vi "Search Text File.vi"(10 "Subject Number":string, 11 "Spreadsheet String":string) -> (0 "SPARC Data":dbl[](array[numeric]), 1 "NMD Data":dbl[](array[numeric]), 2 "SPARC Data Text":string[](array[string]), 3 "NMD Data Text":string[](array[string]))   [LabVIEW 2021]
uses:
  <vilib>/Analysis/baseanly.llb/Mean (DBL).vi
  <vilib>/Analysis/NI_AALBase.lvlib
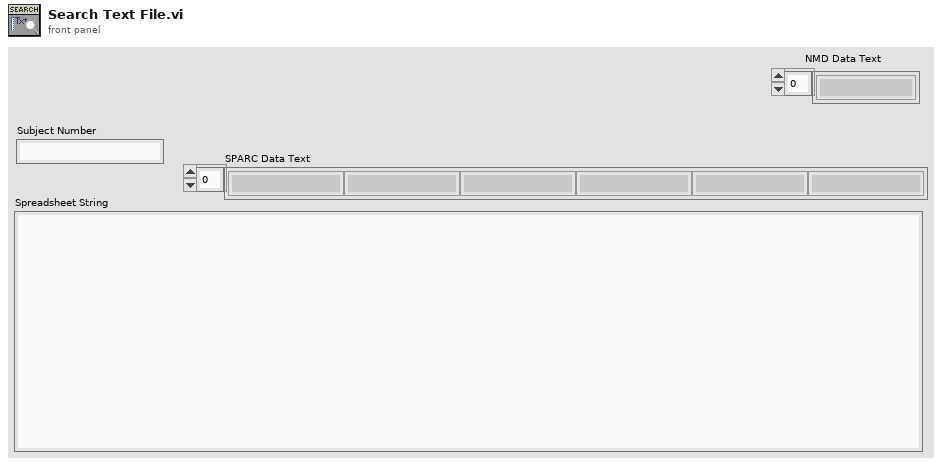
[diagram p1: front panel]
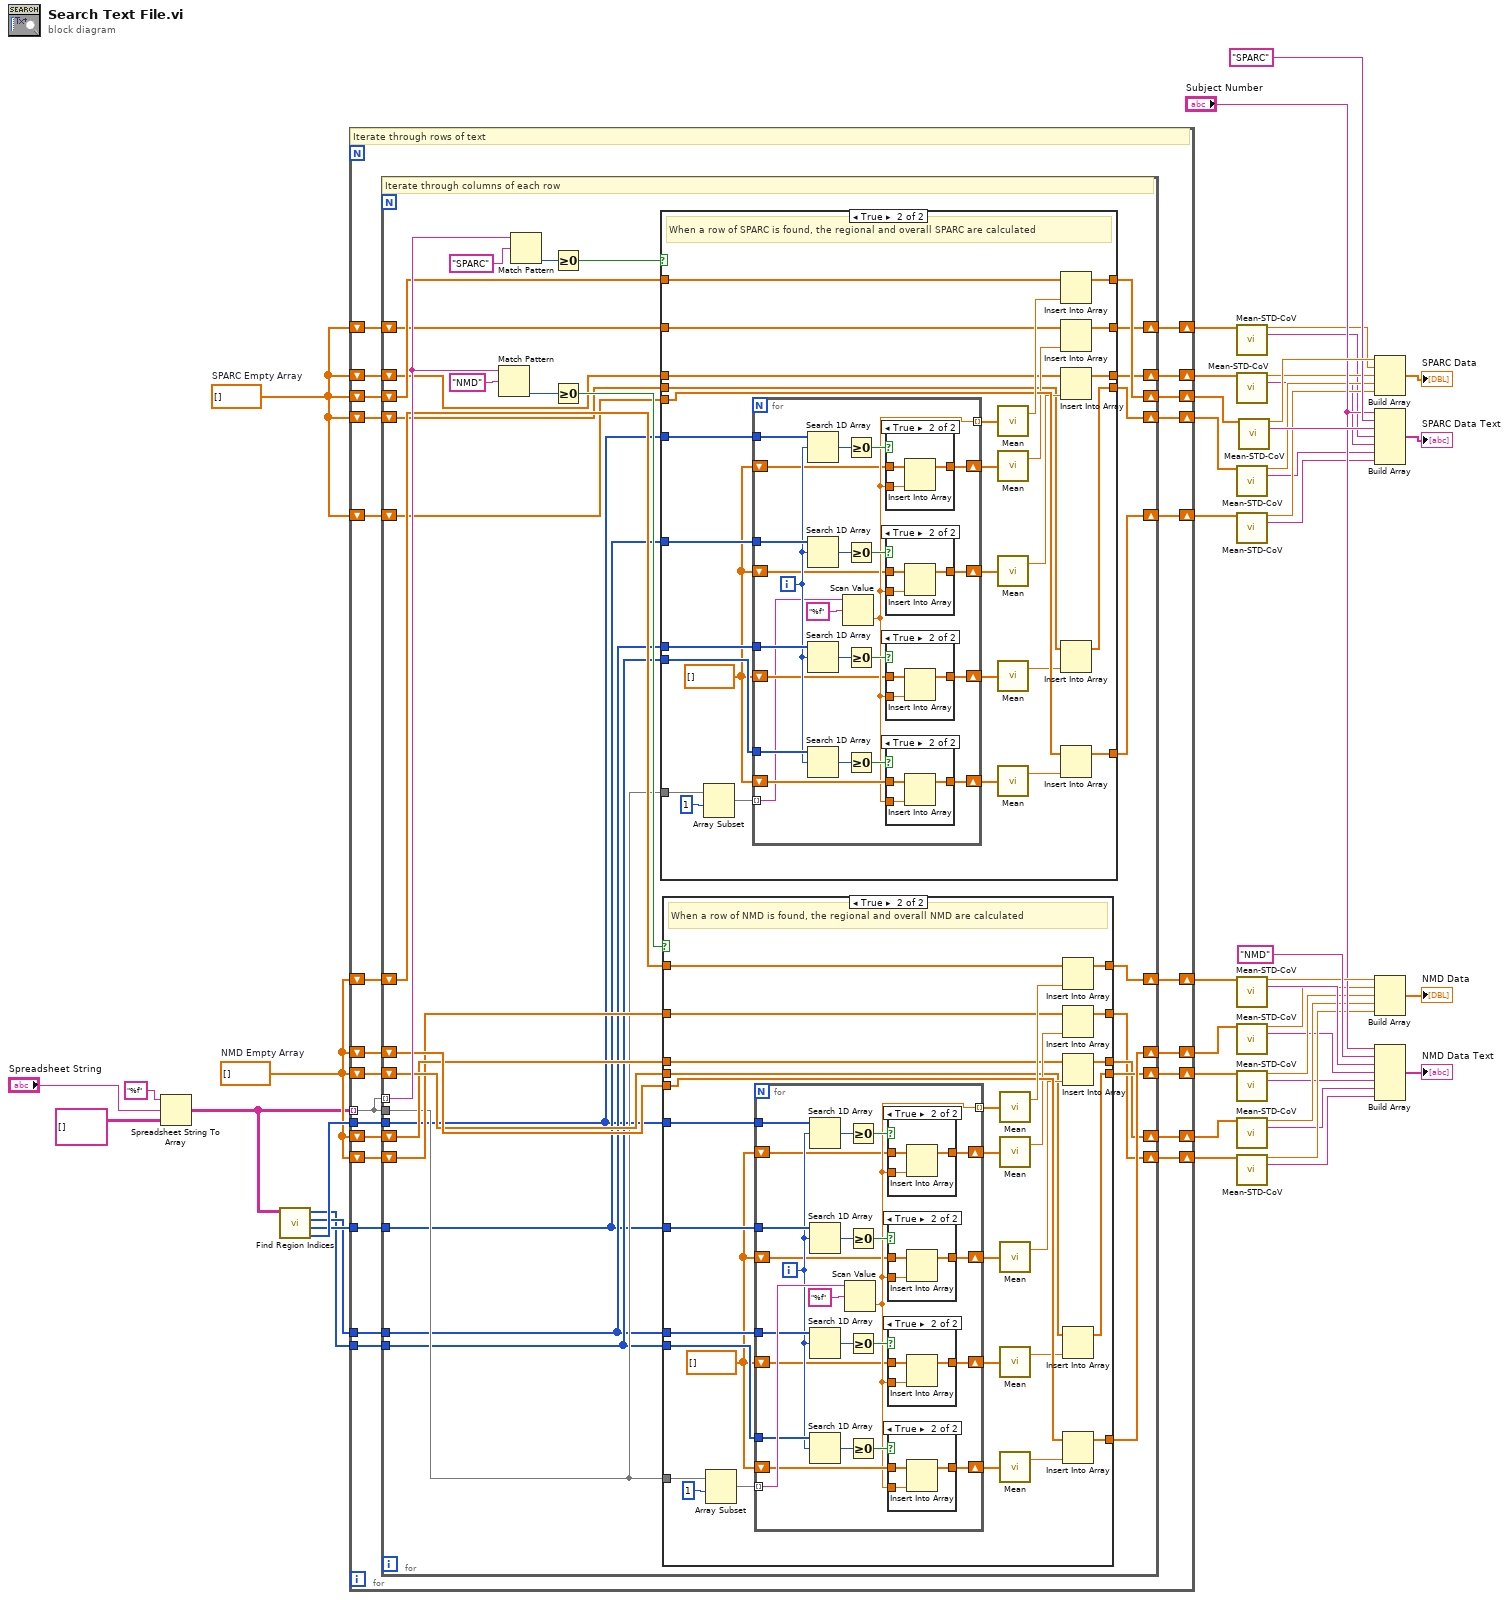
[diagram p0: block diagram]
diagram:
  w38 = dbl[] []  # SPARC Empty Array
  w39 = dbl[] []  # NMD Empty Array
  n1 = Spreadsheet String To Array(format string="%f", spreadsheet string="Spreadsheet String", array type (2D Dbl)=string[][] []) -> (array=w1:string[][])  [unwired: 1 in]
  n2 = call "Find Region Indices.vi"("Spreadsheet Array"=w1) -> ("UES Index"=w43:i32[], "Hypo Index"=w42:i32[], "Tongue Index"=w41:i32[], "Velo Index"=w40:i32[])  [unwired: 7 in]
  n3 = for {
    shift-right: [w71] -> w44
    shift-left: w39 -> [w72]
    shift-right: [w69] -> w31
    shift-left: w38 -> [w70]
    shift-right: [w67] -> w35
    shift-left: w39 -> [w68]
    tunnel: w43 -> [w66]
    tunnel: w42 -> [w65]
    tunnel: w41 -> [w64]
    tunnel: w40 -> [w63]
    tunnel: w1 -> [w62] mode=indexing
    shift-right: [w58] -> w34
    shift-left: w39 -> [w61]
    shift-right: [w57] -> w33
    shift-left: w39 -> [w60]
    shift-right: [w56] -> w32
    shift-left: w39 -> [w59]
    shift-right: [w48] -> w30
    shift-left: w38 -> [w52]
    shift-right: [w49] -> w29
    shift-left: w38 -> [w53]
    shift-right: [w50] -> w28
    shift-left: w38 -> [w54]
    shift-right: [w51] -> w27
    shift-left: w38 -> [w55]
    # "Iterate through rows of text"
    n4 = for {
      tunnel: w62 -> [w100] mode=indexing
      shift-right: [w98] -> w71
      shift-left: w72 -> [w99]
      shift-right: [w82] -> w69
      shift-left: w70 -> [w83]
      shift-right: [w95] -> w67
      shift-left: w68 -> [w96]
      tunnel: w66 -> [w84]
      tunnel: w65 -> [w85]
      tunnel: w64 -> [w86]
      tunnel: w63 -> [w87]
      tunnel: w62 -> [w88]
      shift-right: [w91] -> w58
      shift-left: w61 -> [w94]
      shift-right: [w90] -> w57
      shift-left: w60 -> [w93]
      shift-right: [w89] -> w56
      shift-left: w59 -> [w92]
      shift-right: [w74] -> w48
      shift-left: w52 -> [w78]
      shift-right: [w75] -> w49
      shift-left: w53 -> [w79]
      shift-right: [w76] -> w50
      shift-left: w54 -> [w80]
      shift-right: [w77] -> w51
      shift-left: w55 -> [w81]
      # "Iterate through columns of each row"
      n5 = Match Pattern(string=w100, regular expression="NMD" ("element")) -> (offset past match=w104:i32)  [unwired: 1 in, 3 out]
      n6 = Match Pattern(string=w100, regular expression="SPARC" ("element")) -> (offset past match=w103:i32)  [unwired: 1 in, 3 out]
      n7 = Greater Or Equal To 0?(x=w103) -> (x >= 0?=w73:bool)
      n8 = Greater Or Equal To 0?(x=w104) -> (x >= 0?=w97:bool)
      n9 = case shown="True" w73 {
        tunnel: w83 -> [w109 w135]
        tunnel: [w109 w133] -> w82
        tunnel: w88 -> [_ w132]
        tunnel: w87 -> [_ w131]
        tunnel: w86 -> [_ w128]
        tunnel: w85 -> [_ w129]
        tunnel: w84 -> [_ w130]
        tunnel: w81 -> [w108 w126]
        tunnel: [w108 w125] -> w77
        tunnel: w80 -> [w107 w116]
        tunnel: w79 -> [w106 w115]
        tunnel: w78 -> [w105 w114]
        tunnel: [w107 w113] -> w76
        tunnel: [w106 w112] -> w75
        tunnel: [w105 w111] -> w74
        frame False {
        }
        frame True {
          w123 = dbl[] []
          # "When a row of SPARC is found, the regional and overall SPARC are calculated"
          n10 = Array Subset(array=w132, index=1) -> (w110:string[])  [unwired: 1 in]
          n11 = for {
            tunnel: w110 -> [w138] mode=indexing
            tunnel: [w145] -> w136 mode=indexing
            tunnel: w131 -> [w160]
            tunnel: w130 -> [w159]
            tunnel: w129 -> [w158]
            tunnel: w128 -> [w157]
            shift-right: [w149] -> w127
            shift-left: w123 -> [w150]
            shift-right: [w141] -> w117
            shift-left: w123 -> [w142]
            shift-right: [w140] -> w119
            shift-left: w123 -> [w143]
            shift-right: [w139] -> w121
            shift-left: w123 -> [w144]
            i -> [w152]
            n12 = Search 1D Array(1D array=w159, element=w152) -> (index of element=w154:i32)  [unwired: 1 in]
            n13 = Search 1D Array(1D array=w158, element=w152) -> (index of element=w155:i32)  [unwired: 1 in]
            n14 = Search 1D Array(1D array=w157, element=w152) -> (index of element=w153:i32)  [unwired: 1 in]
            n15 = Search 1D Array(1D array=w160, element=w152) -> (index of element=w156:i32)  [unwired: 1 in]
            n16 = Scan Value(string=w138, format string="%f") -> (value=w145:dbl)  [unwired: 1 in, 1 out]
            n17 = Greater Or Equal To 0?(x=w154) -> (x >= 0?=w146:bool)
            n18 = Greater Or Equal To 0?(x=w155) -> (x >= 0?=w147:bool)
            n19 = Greater Or Equal To 0?(x=w153) -> (x >= 0?=w148:bool)
            n20 = Greater Or Equal To 0?(x=w156) -> (x >= 0?=w151:bool)
            n21 = case shown="True" w146 {
              tunnel: w142 -> [w162 w165]
              tunnel: w145 -> [_ w164]
              tunnel: [w162 w163] -> w141
              frame False {
              }
              frame True {
                n22 = Insert Into Array(array=w165, new element=w164) -> (w163:dbl[])  [unwired: 1 in]
              }
            }
            n23 = case shown="True" w147 {
              tunnel: w143 -> [w166 w169]
              tunnel: w145 -> [_ w168]
              tunnel: [w166 w167] -> w140
              frame False {
              }
              frame True {
                n24 = Insert Into Array(array=w169, new element=w168) -> (w167:dbl[])  [unwired: 1 in]
              }
            }
            n25 = case shown="True" w148 {
              tunnel: w144 -> [w170 w173]
              tunnel: w145 -> [_ w172]
              tunnel: [w170 w171] -> w139
              frame False {
              }
              frame True {
                n26 = Insert Into Array(array=w173, new element=w172) -> (w171:dbl[])  [unwired: 1 in]
              }
            }
            n27 = case shown="True" w151 {
              tunnel: w150 -> [w174 w177]
              tunnel: w145 -> [_ w176]
              tunnel: [w174 w175] -> w149
              frame False {
              }
              frame True {
                n28 = Insert Into Array(array=w177, new element=w176) -> (w175:dbl[])  [unwired: 1 in]
              }
            }
          }
          n29 = call-poly <vilib>:"Mean.vi"("X"=w136) -> ("mean"=w134:dbl)  [unwired: 1 out]
          n30 = call-poly <vilib>:"Mean.vi"("X"=w117) -> ("mean"=w118:dbl)  [unwired: 1 out]
          n31 = call-poly <vilib>:"Mean.vi"("X"=w119) -> ("mean"=w120:dbl)  [unwired: 1 out]
          n32 = call-poly <vilib>:"Mean.vi"("X"=w121) -> ("mean"=w122:dbl)  [unwired: 1 out]
          n33 = call-poly <vilib>:"Mean.vi"("X"=w127) -> ("mean"=w124:dbl)  [unwired: 1 out]
          n34 = Insert Into Array(array=w135, new element=w134) -> (w133:dbl[])  [unwired: 1 in]
          n35 = Insert Into Array(array=w114, new element=w118) -> (w111:dbl[])  [unwired: 1 in]
          n36 = Insert Into Array(array=w115, new element=w120) -> (w112:dbl[])  [unwired: 1 in]
          n37 = Insert Into Array(array=w116, new element=w122) -> (w113:dbl[])  [unwired: 1 in]
          n38 = Insert Into Array(array=w126, new element=w124) -> (w125:dbl[])  [unwired: 1 in]
        }
      }
      n39 = case shown="True" w97 {
        tunnel: w99 -> [w182 w207]
        tunnel: [w182 w205] -> w98
        tunnel: w88 -> [_ w204]
        tunnel: w87 -> [_ w203]
        tunnel: w86 -> [_ w200]
        tunnel: w85 -> [_ w201]
        tunnel: w84 -> [_ w202]
        tunnel: w96 -> [w181 w198]
        tunnel: [w181 w197] -> w95
        tunnel: w94 -> [w180 w188]
        tunnel: w93 -> [w179 w187]
        tunnel: w92 -> [w178 w186]
        tunnel: [w180 w185] -> w91
        tunnel: [w179 w184] -> w90
        tunnel: [w178 w183] -> w89
        frame False {
        }
        frame True {
          w195 = dbl[] []
          # "When a row of NMD is found, the regional and overall NMD are calculated"
          n40 = Array Subset(array=w204, index=1) -> (w209:string[])  [unwired: 1 in]
          n41 = for {
            tunnel: w209 -> [w233] mode=indexing
            tunnel: [w217] -> w208 mode=indexing
            tunnel: w203 -> [w232]
            tunnel: w202 -> [w231]
            tunnel: w201 -> [w230]
            tunnel: w200 -> [w229]
            shift-right: [w221] -> w199
            shift-left: w195 -> [w222]
            shift-right: [w213] -> w189
            shift-left: w195 -> [w214]
            shift-right: [w212] -> w191
            shift-left: w195 -> [w215]
            shift-right: [w211] -> w193
            shift-left: w195 -> [w216]
            i -> [w224]
            n42 = Search 1D Array(1D array=w231, element=w224) -> (index of element=w226:i32)  [unwired: 1 in]
            n43 = Search 1D Array(1D array=w230, element=w224) -> (index of element=w227:i32)  [unwired: 1 in]
            n44 = Search 1D Array(1D array=w229, element=w224) -> (index of element=w225:i32)  [unwired: 1 in]
            n45 = Search 1D Array(1D array=w232, element=w224) -> (index of element=w228:i32)  [unwired: 1 in]
            n46 = Scan Value(string=w233, format string="%f") -> (value=w217:dbl)  [unwired: 1 in, 1 out]
            n47 = Greater Or Equal To 0?(x=w226) -> (x >= 0?=w218:bool)
            n48 = Greater Or Equal To 0?(x=w227) -> (x >= 0?=w219:bool)
            n49 = Greater Or Equal To 0?(x=w225) -> (x >= 0?=w220:bool)
            n50 = Greater Or Equal To 0?(x=w228) -> (x >= 0?=w223:bool)
            n51 = case shown="True" w218 {
              tunnel: w214 -> [w235 w238]
              tunnel: w217 -> [_ w237]
              tunnel: [w235 w236] -> w213
              frame False {
              }
              frame True {
                n52 = Insert Into Array(array=w238, new element=w237) -> (w236:dbl[])  [unwired: 1 in]
              }
            }
            n53 = case shown="True" w219 {
              tunnel: w215 -> [w239 w242]
              tunnel: w217 -> [_ w241]
              tunnel: [w239 w240] -> w212
              frame False {
              }
              frame True {
                n54 = Insert Into Array(array=w242, new element=w241) -> (w240:dbl[])  [unwired: 1 in]
              }
            }
            n55 = case shown="True" w220 {
              tunnel: w216 -> [w243 w246]
              tunnel: w217 -> [_ w245]
              tunnel: [w243 w244] -> w211
              frame False {
              }
              frame True {
                n56 = Insert Into Array(array=w246, new element=w245) -> (w244:dbl[])  [unwired: 1 in]
              }
            }
            n57 = case shown="True" w223 {
              tunnel: w222 -> [w247 w250]
              tunnel: w217 -> [_ w249]
              tunnel: [w247 w248] -> w221
              frame False {
              }
              frame True {
                n58 = Insert Into Array(array=w250, new element=w249) -> (w248:dbl[])  [unwired: 1 in]
              }
            }
          }
          n59 = call-poly <vilib>:"Mean.vi"("X"=w208) -> ("mean"=w206:dbl)  [unwired: 1 out]
          n60 = call-poly <vilib>:"Mean.vi"("X"=w189) -> ("mean"=w190:dbl)  [unwired: 1 out]
          n61 = call-poly <vilib>:"Mean.vi"("X"=w191) -> ("mean"=w192:dbl)  [unwired: 1 out]
          n62 = call-poly <vilib>:"Mean.vi"("X"=w193) -> ("mean"=w194:dbl)  [unwired: 1 out]
          n63 = call-poly <vilib>:"Mean.vi"("X"=w199) -> ("mean"=w196:dbl)  [unwired: 1 out]
          n64 = Insert Into Array(array=w207, new element=w206) -> (w205:dbl[])  [unwired: 1 in]
          n65 = Insert Into Array(array=w186, new element=w190) -> (w183:dbl[])  [unwired: 1 in]
          n66 = Insert Into Array(array=w187, new element=w192) -> (w184:dbl[])  [unwired: 1 in]
          n67 = Insert Into Array(array=w188, new element=w194) -> (w185:dbl[])  [unwired: 1 in]
          n68 = Insert Into Array(array=w198, new element=w196) -> (w197:dbl[])  [unwired: 1 in]
        }
      }
    }
  }
  n69 = call "Mean-STD-CoV.vi"("Data Array"=w30) -> (4:"Mean"=w9:dbl, 6:"Mean"=w5:string)  [unwired: 11 in, 2 out]
  n70 = call "Mean-STD-CoV.vi"("Data Array"=w29) -> (4:"Mean"=w8:dbl, 6:"Mean"=w4:string)  [unwired: 11 in, 2 out]
  n71 = call "Mean-STD-CoV.vi"("Data Array"=w28) -> (4:"Mean"=w7:dbl, 6:"Mean"=w3:string)  [unwired: 11 in, 2 out]
  n72 = call "Mean-STD-CoV.vi"("Data Array"=w27) -> (4:"Mean"=w6:dbl, 6:"Mean"=w2:string)  [unwired: 11 in, 2 out]
  n73 = call "Mean-STD-CoV.vi"("Data Array"=w44) -> (4:"Mean"=w25:dbl, 6:"Mean"=w26:string)  [unwired: 11 in, 2 out]
  n74 = call "Mean-STD-CoV.vi"("Data Array"=w35) -> (4:"Mean"=w17:dbl, 6:"Mean"=w13:string)  [unwired: 11 in, 2 out]
  n75 = call "Mean-STD-CoV.vi"("Data Array"=w34) -> (4:"Mean"=w16:dbl, 6:"Mean"=w12:string)  [unwired: 11 in, 2 out]
  n76 = call "Mean-STD-CoV.vi"("Data Array"=w33) -> (4:"Mean"=w15:dbl, 6:"Mean"=w11:string)  [unwired: 11 in, 2 out]
  n77 = call "Mean-STD-CoV.vi"("Data Array"=w32) -> (4:"Mean"=w14:dbl, 6:"Mean"=w10:string)  [unwired: 11 in, 2 out]
  n78 = call "Mean-STD-CoV.vi"("Data Array"=w31) -> (4:"Mean"=w22:dbl, 6:"Mean"=w19:string)  [unwired: 11 in, 2 out]
  n79 = Build Array(w22, w9, w8, w7, w6) -> (→"SPARC Data":dbl[])
  n80 = Build Array("Subject Number", "SPARC" ("element"), w19, w5, w4, w3, w2) -> (→"SPARC Data Text":string[])
  n81 = Build Array(w25, w17, w16, w15, w14) -> (→"NMD Data":dbl[])
  n82 = Build Array("Subject Number", "NMD" ("element"), w26, w13, w12, w11, w10) -> (→"NMD Data Text":string[])
